vi "5.10.Larry Steering.vi"(1 "Certainty of Line (High is more certain scale is arbitrary)":dbl) -> (0 "Numeric":dbl)   [LabVIEW 2011]
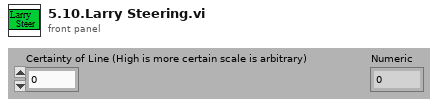
[diagram p1: front panel]
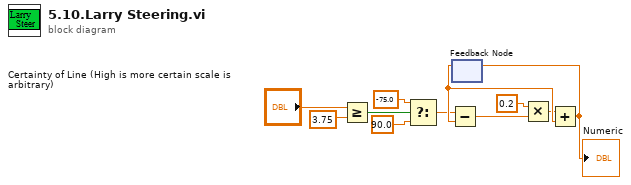
[diagram p0: block diagram]
diagram:
  n1 = Greater Or Equal?(x="Certainty of Line (High is more certain scale is arbitrary)", y=3.75) -> (x >= y?=w11:bool)
  n2 = Select(t=-75.0, s=w11, f=90.0) -> (s? t:f=w5:dbl)
  n3 = feedback #1() -> (w10:dbl)  [unwired: 1 in]
  n4 = Subtract(x=w5, y=w10) -> (x-y=w6:dbl)
  n5 = Multiply(x=0.2, y=w6) -> (x*y=w8:dbl)
  n6 = Add(x=w8, y=w10) -> (x+y=w9:dbl)
  "Numeric" <- w9
  n7 = feedback-in #1(w9) -> ()
